vi "Run Assert Display.vi"   [LabVIEW 2016, in "Assert API Components.lvlib"]
uses:
  Assert API Components/Assert API Components.lvlib
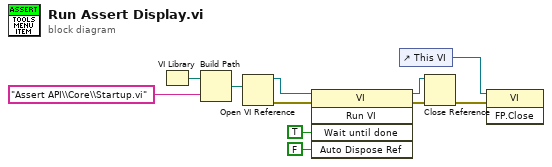
[diagram p0: block diagram]
diagram:
  n1 = VI Library() -> (path=w11:path)
  n2 = Build Path(base path=w11, name or relative path="Assert API\\Core\\Startup.vi") -> (appended path=w9:path)
  n3 = Open VI Reference(vi path=w9) -> (vi reference=w8:refnum<vi>, error out=w7:errorcluster)  [unwired: 5 in]
  n4 = invoke class="VI" method="Run VI"(reference=w8, error in=w7, "Wait until done"=TRUE ("Wait Until Done"), "Auto Dispose Ref"=FALSE ("Auto Dispose Reference")) -> (reference out=w6:refnum<vi>, error out=w5:errorcluster)  [unwired: 1 in, 3 out]
  n5 = control-ref of="This VI"() -> (w3:refnum<vi>)
  n6 = Close Reference(reference=w6, error in (no error)=w5) -> (error out=w4:errorcluster)
  n7 = invoke class="VI" method="FP.Close"(reference=w3, error in=w4) -> ()  [unwired: 1 in, 3 out]
